vi "WorkorderHandler_GetOrderList.vi"(8 "error in (no error)":errorcluster, 10 "Script":string, 11 "reference":T1) -> (0 "error out":errorcluster, 2 "Orders":string[](array[string]), 3 "duplicate reference":T1)   [LabVIEW 2011]
uses:
  DataStructures/WorkorderHandler_ObjectReference.ctl
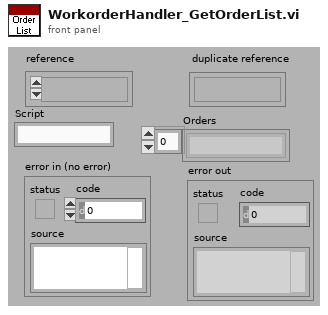
[diagram p1: front panel]
types:
  T1 = typedef "WorkorderHandler_ObjectReference.ctl" = refnum<k1>
  T2 = typedef "WorkorderHandler_ObjectData.ctl" = cluster{"Table":string[][], "Script":string, "Order":string, "No":string, "Time":dbl}
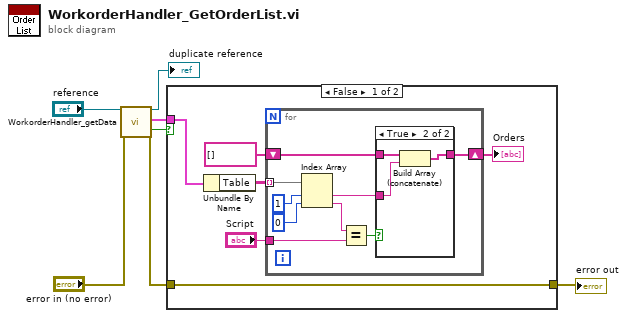
[diagram p0: block diagram]
diagram:
  n1 = call "WorkorderHandler_getData.vi"("reference"="reference", "error in (no error)"="error in (no error)") -> ("duplicate reference"=→"duplicate reference":T1, "data"=w5:T2, "timed out?"=w1:bool, "error out"=w2:errorcluster)  [unwired: 1 in, 13 out]
  n2 = case shown="False" w1 {
    tunnel: w5 -> [w13 _]
    tunnel: [w12 w27] -> w4
    tunnel: w2 -> [w12 w27]
    frame False {
      n3 = Unbundle By Name(w13) -> ("Table"=w11:string[][])
      n4 = for {
        tunnel: w11 -> [w22] mode=indexing
        tunnel: "Script" -> [w18]
        shift-right: [w14] -> w9
        shift-left: string[] [] -> [w15]
        n5 = Index Array(array=w22, index #1=1 ("index"), index #2=0 ("index")) -> (element #1=w16:string, element #2=w19:string)
        n6 = Equal?(x=w19, y=w18) -> (x = y?=w17:bool)
        n7 = case shown="True" w17 {
          tunnel: w16 -> [_ w26]
          tunnel: w15 -> [w23 w25]
          tunnel: [w23 w24] -> w14
          frame False {
          }
          frame True {
            n8 = Build Array (concatenate)(w25, w26) -> (w24:string[])
          }
        }
      }
      "Orders" <- w9
    }
    frame True {
      # "Error or Timed Out"
    }
  }
  "error out" <- w4
